vi "WILT Turn Water Valve On.vi"(4 "Day/Night Cycle":T1, 5 "Valve Status":T4, 6 "Semaphore":T2[](array[typedef]), 7 "Station Group":T3, 8 "error in (no error)":errorcluster, 9 "Agilent Valve and Switch Locations":T5[](array[typedef])=[{"Channel"="301", "Station"="1", "Label"="Water Valve", "Agilent Station"="2", "Data"=0.0}, {"Channel"="302", "Station"="2", "Label"="Water Valve", "Agilent Station"="2", "Data"=0.0}, {"Channel"="303", "Station"="3", "Label"="Water Valve", "Agilent Station"="2", "Data"=0.0}, {"Channel"="304", "Station"="4", "Label"="Water Valve", "Agilent Station"="2", "Data"=0.0}, {"Channel"="305", "Station"="5", "Label"="Water Valve", "Agilent Station"="2", "Data"=0.0}, {"Channel"="306", "Station"="6", "Label"="Water Valve", "Agilent Station"="2", "Data"=0.0}, {"Channel"="307", "Station"="7", "Label"="Water Valve", "Agilent Station"="2", "Data"=0.0}, {"Channel"="308", "Station"="8", "Label"="Water Valve", "Agilent Station"="2", "Data"=0.0}, {"Channel"="309", "Station"="9", "Label"="Water Valve", "Agilent Station"="2", "Data"=0.0}, {"Channel"="310", "Station"="10", "Label"="Water Valve", "Agilent Station"="2", "Data"=0.0}, {"Channel"="311", "Station"="11", "Label"="Water Valve", "Agilent Station"="2", "Data"=0.0}, {"Channel"="312", "Station"="12", "Label"="Water Valve", "Agilent Station"="2", "Data"=0.0}, {"Channel"="313", "Station"="13", "Label"="Water Valve", "Agilent Station"="2", "Data"=0.0}, {"Channel"="314", "Station"="14", "Label"="Water Valve", "Agilent Station"="2", "Data"=0.0}, {"Channel"="315", "Station"="15", "Label"="Water Valve", "Agilent Station"="2", "Data"=0.0}, {"Channel"="316", "Station"="16", "Label"="Water Valve", "Agilent Station"="2", "Data"=0.0}, {"Channel"="317", "Station"="17", "Label"="Water Valve", "Agilent Station"="2", "Data"=0.0}, {"Channel"="318", "Station"="18", "Label"="Water Valve", "Agilent Station"="2", "Data"=0.0}, {"Channel"="319", "Station"="19", "Label"="Water Valve", "Agilent Station"="2", "Data"=0.0}, {"Channel"="320", "Station"="20", "Label"="Water Valve", "Agilent Station"="2", "Data"=0.0}, {"Channel"="101", "Station"="21", "Label"="Water Valve", "Agilent Station"="3", "Data"=0.0}, {"Channel"="102", "Station"="22", "Label"="Water Valve", "Agilent Station"="3", "Data"=0.0}, {"Channel"="103", "Station"="23", "Label"="Water Valve", "Agilent Station"="3", "Data"=0.0}, {"Channel"="104", "Station"="24", "Label"="Water Valve", "Agilent Station"="3", "Data"=0.0}, {"Channel"="105", "Station"="25", "Label"="Water Valve", "Agilent Station"="3", "Data"=0.0}, {"Channel"="106", "Station"="26", "Label"="Water Valve", "Agilent Station"="3", "Data"=0.0}, {"Channel"="107", "Station"="27", "Label"="Water Valve", "Agilent Station"="3", "Data"=0.0}, {"Channel"="108", "Station"="28", "Label"="Water Valve", "Agilent Station"="3", "Data"=0.0}, {"Channel"="109", "Station"="29", "Label"="Water Valve", "Agilent Station"="3", "Data"=0.0}, {"Channel"="110", "Station"="30", "Label"="Water Valve", "Agilent Station"="3", "Data"=0.0}, {"Channel"="111", "Station"="31", "Label"="Water Valve", "Agilent Station"="3", "Data"=0.0}, {"Channel"="112", "Station"="32", "Label"="Water Valve", "Agilent Station"="3", "Data"=0.0}, {"Channel"="101", "Station"="33", "Label"="Water Valve", "Agilent Station"="5", "Data"=0.0}, {"Channel"="102", "Station"="34", "Label"="Water Valve", "Agilent Station"="5", "Data"=0.0}, {"Channel"="103", "Station"="35", "Label"="Water Valve", "Agilent Station"="5", "Data"=0.0}, {"Channel"="104", "Station"="36", "Label"="Water Valve", "Agilent Station"="5", "Data"=0.0}, {"Channel"="105", "Station"="37", "Label"="Water Valve", "Agilent Station"="5", "Data"=0.0}, {"Channel"="106", "Station"="38", "Label"="Water Valve", "Agilent Station"="5", "Data"=0.0}, {"Channel"="107", "Station"="39", "Label"="Water Valve", "Agilent Station"="5", "Data"=0.0}, {"Channel"="108", "Station"="40", "Label"="Water Valve", "Agilent Station"="5", "Data"=0.0}, {"Channel"="109", "Station"="41", "Label"="Water Valve", "Agilent Station"="5", "Data"=0.0}, {"Channel"="110", "Station"="42", "Label"="Water Valve", "Agilent Station"="5", "Data"=0.0}, {"Channel"="111", "Station"="43", "Label"="Water Valve", "Agilent Station"="5", "Data"=0.0}, {"Channel"="112", "Station"="44", "Label"="Water Valve", "Agilent Station"="5", "Data"=0.0}, {"Channel"="113", "Station"="45", "Label"="Water Valve", "Agilent Station"="5", "Data"=0.0}, {"Channel"="114", "Station"="46", "Label"="Water Valve", "Agilent Station"="5", "Data"=0.0}, {"Channel"="115", "Station"="47", "Label"="Water Valve", "Agilent Station"="5", "Data"=0.0}, {"Channel"="116", "Station"="48", "Label"="Water Valve", "Agilent Station"="5", "Data"=0.0}, {"Channel"="117", "Station"="49", "Label"="Water Valve", "Agilent Station"="5", "Data"=0.0}, {"Channel"="118", "Station"="50", "Label"="Water Valve", "Agilent Station"="5", "Data"=0.0}, {"Channel"="119", "Station"="51", "Label"="Water Valve", "Agilent Station"="5", "Data"=0.0}, {"Channel"="120", "Station"="52", "Label"="Water Valve", "Agilent Station"="5", "Data"=0.0}, {"Channel"="201", "Station"="53", "Label"="Water Valve", "Agilent Station"="5", "Data"=0.0}, {"Channel"="202", "Station"="54", "Label"="Water Valve", "Agilent Station"="5", "Data"=0.0}, {"Channel"="203", "Station"="55", "Label"="Water Valve", "Agilent Station"="5", "Data"=0.0}, {"Channel"="204", "Station"="56", "Label"="Water Valve", "Agilent Station"="5", "Data"=0.0}, {"Channel"="301", "Station"="21", "Label"="Start Button", "Agilent Station"="5", "Data"=0.0}, {"Channel"="302", "Station"="22", "Label"="Start Button", "Agilent Station"="5", "Data"=0.0}, {"Channel"="303", "Station"="23", "Label"="Start Button", "Agilent Station"="5", "Data"=0.0}, {"Channel"="304", "Station"="24", "Label"="Start Button", "Agilent Station"="5", "Data"=0.0}, {"Channel"="305", "Station"="25", "Label"="Start Button", "Agilent Station"="5", "Data"=0.0}, {"Channel"="306", "Station"="26", "Label"="Start Button", "Agilent Station"="5", "Data"=0.0}, {"Channel"="307", "Station"="27", "Label"="Start Button", "Agilent Station"="5", "Data"=0.0}, {"Channel"="308", "Station"="28", "Label"="Start Button", "Agilent Station"="5", "Data"=0.0}, {"Channel"="309", "Station"="29", "Label"="Start Button", "Agilent Station"="5", "Data"=0.0}, {"Channel"="310", "Station"="30", "Label"="Start Button", "Agilent Station"="5", "Data"=0.0}, {"Channel"="311", "Station"="31", "Label"="Start Button", "Agilent Station"="5", "Data"=0.0}, {"Channel"="312", "Station"="32", "Label"="Start Button", "Agilent Station"="5", "Data"=0.0}, {"Channel"="101", "Station"="33", "Label"="Start Button", "Agilent Station"="7", "Data"=0.0}, {"Channel"="102", "Station"="34", "Label"="Start Button", "Agilent Station"="7", "Data"=0.0}, {"Channel"="103", "Station"="35", "Label"="Start Button", "Agilent Station"="7", "Data"=0.0}, {"Channel"="104", "Station"="36", "Label"="Start Button", "Agilent Station"="7", "Data"=0.0}, {"Channel"="105", "Station"="37", "Label"="Start Button", "Agilent Station"="7", "Data"=0.0}, {"Channel"="106", "Station"="38", "Label"="Start Button", "Agilent Station"="7", "Data"=0.0}, {"Channel"="107", "Station"="39", "Label"="Start Button", "Agilent Station"="7", "Data"=0.0}, {"Channel"="108", "Station"="40", "Label"="Start Button", "Agilent Station"="7", "Data"=0.0}, {"Channel"="109", "Station"="41", "Label"="Start Button", "Agilent Station"="7", "Data"=0.0}, {"Channel"="110", "Station"="42", "Label"="Start Button", "Agilent Station"="7", "Data"=0.0}, {"Channel"="111", "Station"="43", "Label"="Start Button", "Agilent Station"="7", "Data"=0.0}, {"Channel"="112", "Station"="44", "Label"="Start Button", "Agilent Station"="7", "Data"=0.0}, {"Channel"="113", "Station"="45", "Label"="Start Button", "Agilent Station"="7", "Data"=0.0}, {"Channel"="114", "Station"="46", "Label"="Start Button", "Agilent Station"="7", "Data"=0.0}, {"Channel"="115", "Station"="47", "Label"="Start Button", "Agilent Station"="7", "Data"=0.0}, {"Channel"="116", "Station"="48", "Label"="Start Button", "Agilent Station"="7", "Data"=0.0}, {"Channel"="117", "Station"="49", "Label"="Start Button", "Agilent Station"="7", "Data"=0.0}, {"Channel"="118", "Station"="50", "Label"="Start Button", "Agilent Station"="7", "Data"=0.0}, {"Channel"="119", "Station"="51", "Label"="Start Button", "Agilent Station"="7", "Data"=0.0}, {"Channel"="120", "Station"="52", "Label"="Start Button", "Agilent Station"="7", "Data"=0.0}, {"Channel"="201", "Station"="53", "Label"="Start Button", "Agilent Station"="7", "Data"=0.0}, {"Channel"="202", "Station"="54", "Label"="Start Button", "Agilent Station"="7", "Data"=0.0}, {"Channel"="203", "Station"="55", "Label"="Start Button", "Agilent Station"="7", "Data"=0.0}, {"Channel"="204", "Station"="56", "Label"="Start Button", "Agilent Station"="7", "Data"=0.0}], 10 "Station Index":u32, 11 "USB6008":tag) -> (0 "error out":errorcluster)   [LabVIEW 2016]
uses:
  Type Definitions/WILT Agilent Channel Definition.ctl
  Type Definitions/WILT Water Valve Control.ctl
  Type Definitions/WILT Room Location.ctl
  Type Definitions/WILT Day Night Cycle Enum.ctl
  Type Definitions/WILT Water Valve Test Type.ctl
  Type Definitions/WILT Switch Search.ctl
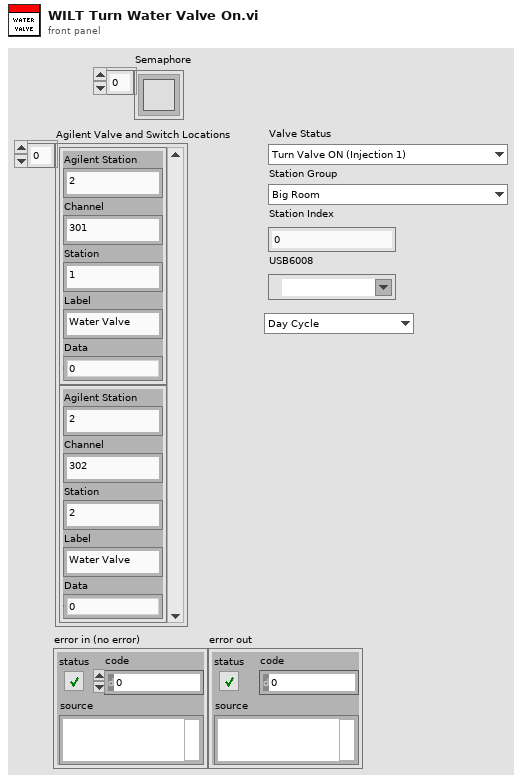
[diagram p1: front panel]
types:
  T1 = typedef "WILT Day Night Cycle Enum.ctl" = enum16{"Day Cycle", "Night Cycle", "Day Cycle (No Water)"}
  T2 = typedef "Semaphore RefNum" = refnum<k1>
  T3 = typedef "WILT Room Location.ctl" = enum16{"Big Room", "Remote Stations"}
  T4 = typedef "WILT Water Valve Control.ctl" = enum16{"Turn Valve ON (Injection 1)", "Turn Valve OFF (Injection 1)", "Turn Valve ON (Injection 2)", "Turn Valve OFF (Injection 2)"}
  T5 = typedef "WILT Agilent Channel Definition.ctl" = cluster{"Channel":string, "Station":string, "Label":string, "Agilent Station":string, "Data":dbl}
  T6 = typedef "WILT Switch Search.ctl" = string
  T7 = typedef "WILT Water Valve Test Type.ctl" = enum16{"Cycle Valve Control", "Full Valve Control"}
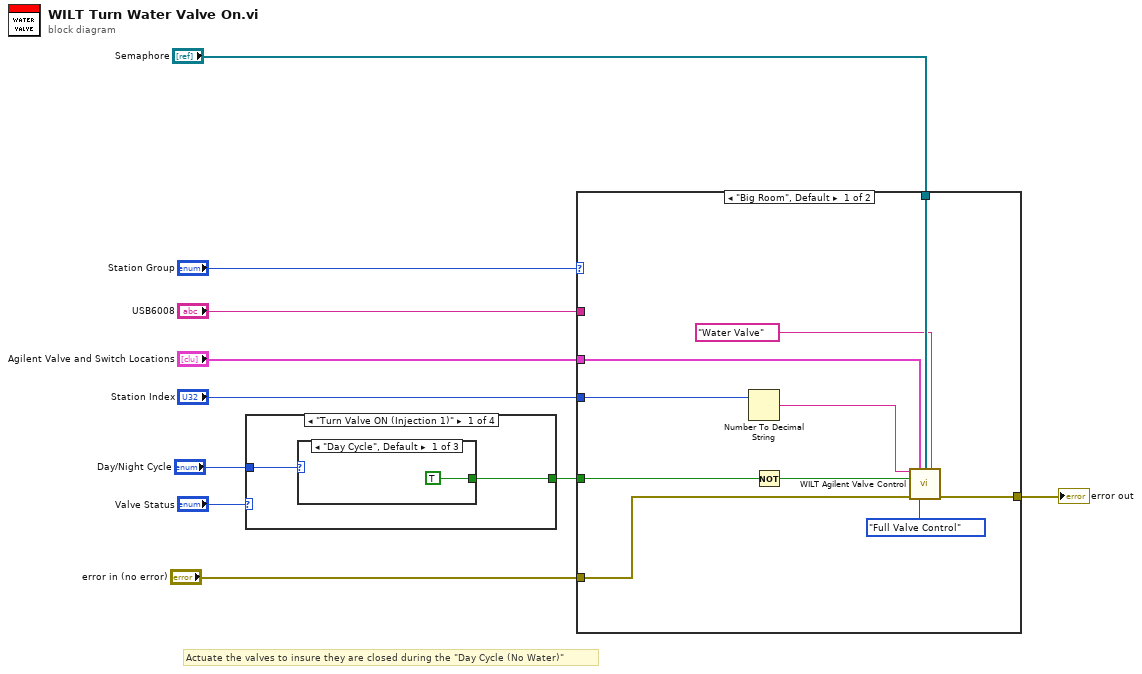
[diagram p0: block diagram]
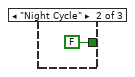
[diagram p2: hidden frame]
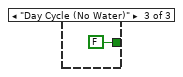
[diagram p3: hidden frame]
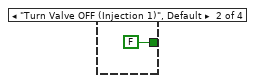
[diagram p4: hidden frame]
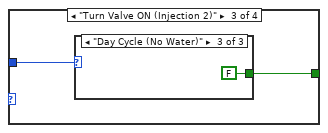
[diagram p5: hidden frame]
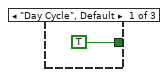
[diagram p6: hidden frame]
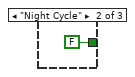
[diagram p7: hidden frame]
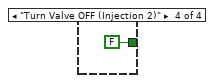
[diagram p8: hidden frame]
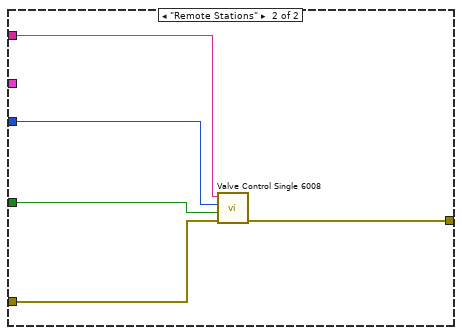
[diagram p9: hidden frame]
diagram:
  # "Actuate the valves to insure they are closed during the \"Day Cycle (No Water)\""
  n1 = case shown="\"Turn Valve ON (Injection 1)\"" "Valve Status" {
    tunnel: [w12 FALSE w18 FALSE] -> w6
    tunnel: "Day/Night Cycle" -> [w11 _ w17 _]
    frame "Turn Valve ON (Injection 1)" {
      n2 = case shown="\"Day Cycle\", Default" w11 {
        tunnel: [TRUE FALSE FALSE] -> w12
        frame "Day Cycle", Default {
        }
        frame "Night Cycle" {
        }
        frame "Day Cycle (No Water)" {
        }
      }
    }
    frame "Turn Valve OFF (Injection 1)", Default {
    }
    frame "Turn Valve ON (Injection 2)" {
      n3 = case shown="\"Day Cycle (No Water)\"" w17 {
        tunnel: [TRUE FALSE FALSE] -> w18
        frame "Day Cycle", Default {
        }
        frame "Night Cycle" {
        }
        frame "Day Cycle (No Water)" {
        }
      }
    }
    frame "Turn Valve OFF (Injection 2)" {
    }
  }
  n4 = case shown="\"Big Room\", Default" "Station Group" {
    tunnel: "Station Index" -> [w28 w36]
    tunnel: "error in (no error)" -> [w32 w34]
    tunnel: "Agilent Valve and Switch Locations" -> [w31 _]
    tunnel: [w30 w33] -> w8
    tunnel: "USB6008" -> [_ w37]
    tunnel: w6 -> [w26 w35]
    tunnel: "Semaphore" -> [w25 _]
    frame "Big Room", Default {
      n5 = Number To Decimal String(number=w28) -> (decimal integer string=w27:string)  [unwired: 1 in]
      n6 = Not(x=w26) -> (.not. x?=w29:bool)
      n7 = call "WILT Agilent Valve Control.vi"("Station In"=w27, "Agilent Channels In"=w31, "Semaphore"=w25, "Search"=T6 "Water Valve", "Open/Close (F:Close)"=w29, "error in (no error)"=w32, "Test Type"=WILT_Water_Valve_Test_Type."Full Valve Control") -> ("error out"=w30:errorcluster)  [unwired: 6 in, 2 out]
    }
    frame "Remote Stations" {
      n8 = call "Valve Control Single 6008.vi"("error in"=w34, "Valve On?"=w35, "Valve Number"=w36, "Port"=w37) -> ("error out"=w33:errorcluster)  [unwired: 7 in]
    }
  }
  "error out" <- w8
